vi "setPosition.vi"(8 "error in (no error)":errorcluster, 9 "Y Position":i32, 10 "X Position":i32, 11 "Stimulus in":refnum<class "Stimulus.lvclass">) -> (0 "error out":errorcluster, 3 "Stimulus out":refnum<class "Stimulus.lvclass">)   [LabVIEW 2013]
uses:
  Stimulus.lvclass
panel:
  in  "index":i32
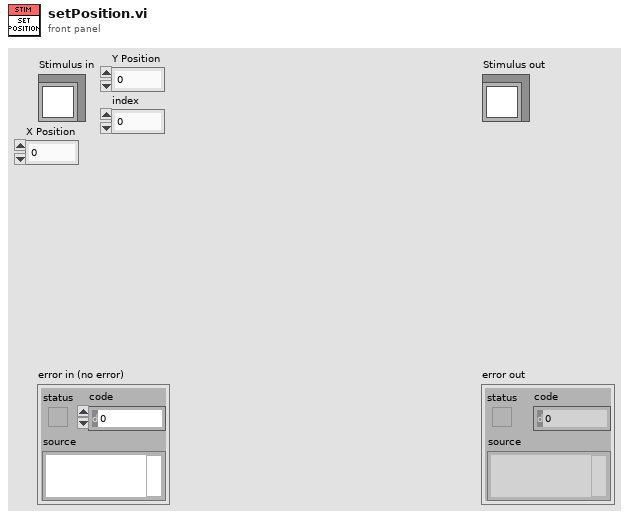
[diagram p1: front panel]
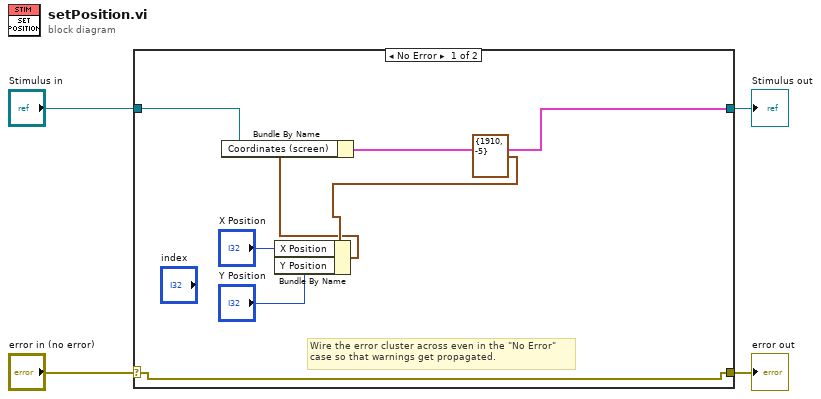
[diagram p0: block diagram]
diagram:
  n1 = case shown="No Error" "error in (no error)" {
    selector: "error in (no error)" -> [w8 w13]
    tunnel: [w8 w13] -> w3
    tunnel: [w5 w12] -> w1
    tunnel: "Stimulus in" -> [w7 w12]
    frame No Error {
      # "Wire the error cluster across even in the \"No Error\"\ncase so that warnings get propagated."
      n2 = Bundle By Name(cluster=cluster{"X Position":i32, "Y Position":i32} {"X Position"=1910, "Y Position"=-5} ("Coordinates (screen)"), "X Position"="X Position", "Y Position"="Y Position") -> (w6:cluster{"X Position":i32, "Y Position":i32})
      n3 = Bundle By Name(cluster=w7, "Coordinates (screen)"=w6) -> (w5:cluster{})
    }
    frame Error {
    }
  }
  "error out" <- w3
  "Stimulus out" <- w1
